vi "Write LogFile Path.vi"(6 "Procedure Type":enum16{"Potting", "Gluing"}(ring), 8 "error in":errorcluster, 10 "LogFile Directory":path, 11 "Console Log in":refnum<class "Console Log.lvclass">) -> (0 "error out":errorcluster, 3 "Console Log out":refnum<class "Console Log.lvclass">)   [LabVIEW 2011, in "Console Log.lvclass"]
uses:
  Console Log.lvclass
  Console Log.lvclass/Console Log.ctl
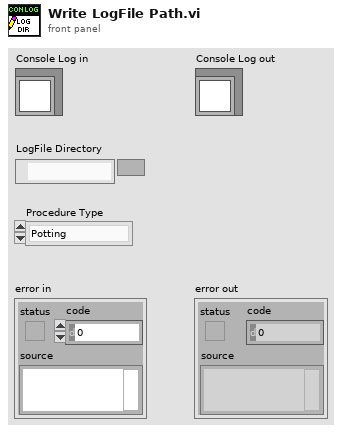
[diagram p1: front panel]
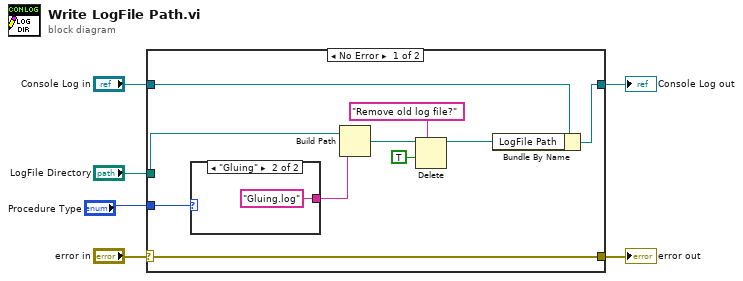
[diagram p0: block diagram]
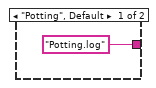
[diagram p2: hidden frame]
diagram:
  n1 = case shown="No Error" "error in" {
    selector: "error in" -> [w16 w19]
    tunnel: [w16 w19] -> w5
    tunnel: [w14 w20] -> w3
    tunnel: "Console Log in" -> [w15 w20]
    tunnel: "LogFile Directory" -> [w13 _]
    tunnel: "Procedure Type" -> [w7 _]
    frame No Error {
      n2 = case shown="\"Gluing\"" w7 {
        tunnel: ["Potting.log" ("time format string (%c)") "Gluing.log" ("time format string (%c)")] -> w12
        frame "Potting", Default {
        }
        frame "Gluing" {
        }
      }
      n3 = Build Path(base path=w13, name or relative path=w12) -> (appended path=w11:path)
      n4 = Delete(prompt (Delete)="Remove old log file?", path (use dialog)=w11, confirm (F)=TRUE) -> (deleted path=w10:path)  [unwired: 2 in, 2 out]
      n5 = Bundle By Name(cluster=w15, "LogFile Path"=w10) -> (w14:refnum<class "Console Log.lvclass">)
    }
    frame Error {
    }
  }
  "error out" <- w5
  "Console Log out" <- w3
